vi "REV Color Sensor.vi"() -> ()   [LabVIEW 2019]
doc: "This example shows how to use the SRF08 Ultrasonic Range Finder via the I2C bus. It can display the distance from the sensor in inches or centimeters.\n\nThis example expects a USB cable connected from your development PC to the Type B USB Jack (next to the power input) on the roboRIO."
uses:
  <vilib>/Rock Robotics/SystemInterfaces/i2clib/i2c_bus.ctl
  <vilib>/Rock Robotics/WPI/Ultrasonic/WPI_SonarSRF08DeviceAddress.ctl
  <vilib>/Rock Robotics/WPI/Ultrasonic/WPI_SonarSRF08_I2C_Close.vi
panel:
  out "Normalized Color":cluster{"R":dbl, "G":dbl, "B":dbl}
  out "Color":u32(colorbox)
  in  "Device Address":T1=224 items=["Dev 0"=224, "Dev 1"=226, "Dev 2"=228, "Dev 3"=230, "Dev 4"=232, "Dev 5"=234, "Dev 6"=236, "Dev 7"=238, "Dev 8"=240, "Dev 9"=242, "Dev 10"=244, "Dev 11"=246, "Dev 12"=248, "Dev 13"=250, "Dev 14"=252, "Dev 15"=254]
  in  "I2C Bus":T2
  in  "stop":bool
  # "Set these inputs before running."
  # "This can be set while running."
  # "Output information."
  # "This shows wiring for the SRF08 ultrasonic range finder.\nNote the I2C header provides 3.3V, so this sensor gets its 5V power from the 5V rail - in this case DIO-0."
  # "SRF08\nGnd (black wire)------\nPower (red wire)------\nSCL (yellow wire)-----\nSDA (white wire)------"
  # "roboRIO\nI2C  \nDIO0   V\nI2C   SCL\nI2C   SDA"
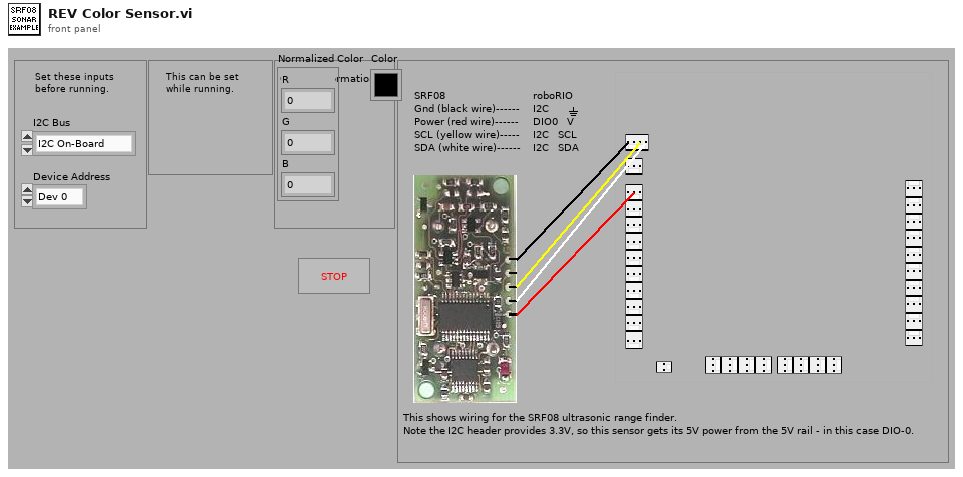
[diagram p1: front panel]
types:
  T1 = typedef "WPI_SonarSRF08DeviceAddress.ctl" = u8
  T2 = typedef "i2c_bus.ctl" = enum16{"I2C On-Board", "I2C MXP", "Invalid"}
  T3 = typedef "Color Sensor V3 DevRef.ctl" = cluster{"I2CDevRef":T4}
  T4 = typedef "WPI_I2CDevRef.ctl" = cluster{"DevStatus":errorcluster, "Device Address":u8, "Handle":i32, "I2C Bus":T2}
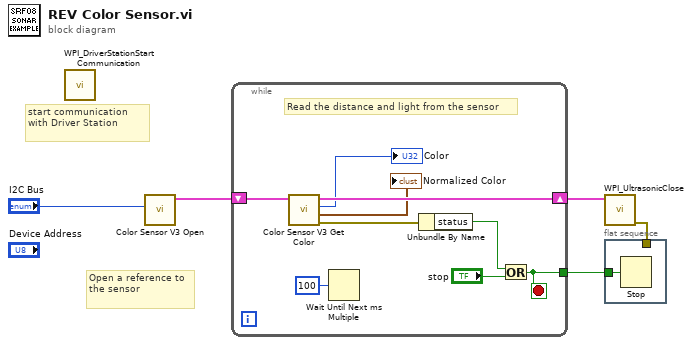
[diagram p0: block diagram]
diagram:
  # "start communication with Driver Station"
  # "Open a reference to the sensor"
  n1 = call <vilib>:"WPI_DriverStationStart Communication.vi"() -> ()  [unwired: 2 in, 10 out]
  n2 = call <vilib>:"Color Sensor V3 Open.vi"("I2C Bus"="I2C Bus") -> ("ColorSensorDevRef"=w1:T3)  [unwired: 9 in, 1 out]
  n3 = while {
    tunnel: [w12] -> w5
    shift-right: [w8] -> w4
    shift-left: w1 -> [w9]
    stop <- w12 stop-if-true
    # "Read the distance and light from the sensor"
    n4 = call <vilib>:"Color Sensor V3 Get Color.vi"("ColorSensorDevRef"=w9) -> ("error out"=w10:errorcluster, "Normalized Color"=→"Normalized Color":cluster{"R":dbl, "G":dbl, "B":dbl}, "Color"=→"Color":u32, "ColorSensorDevRef out"=w8:T3)  [unwired: 7 in]
    n5 = Wait Until Next ms Multiple(millisecond multiple=u32 100 ("milliseconds to wait")) -> ()  [unwired: 1 out]
    n6 = Unbundle By Name(w10) -> ("status"=w14:bool)
    n7 = Or(x=w14, y="stop") -> (x .or. y?=w12:bool)
  }
  n8 = call-poly <vilib>:"WPI_UltrasonicClose.vi"("SonarSRF08_I2C_DevRef"=w4) -> ("error out"=w3:errorcluster)  [unwired: 10 in]
  n9 = flat-sequence {
    tunnel: w5 -> [w15]
    tunnel: w3 -> [_]
    frame #0 {
      n10 = Stop(stop? (T)=w15) -> ()
    }
  }
